vi "HRM-AQN-simulated_read.vi"(8 "error in (no error)":errorcluster, 11 "AQN cluster in":T1) -> (0 "error out":errorcluster, 2 "data":waveform(dbl), 3 "AQN cluster out":T1)   [LabVIEW 2020]
uses:
  HRM-AQN-input_clust.ctl
  <vilib>/measure/NI_MABase.lvlib
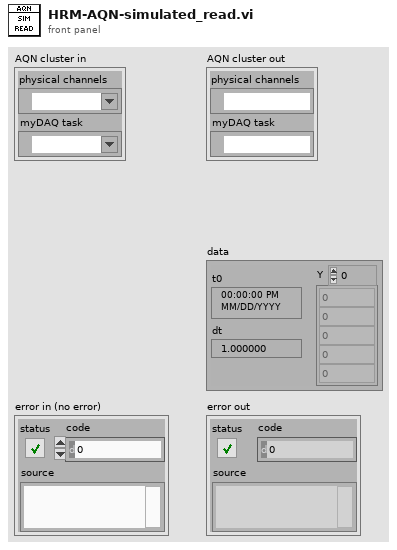
[diagram p1: front panel]
types:
  T1 = typedef "HRM-AQN-input_clust.ctl" = cluster{"physical channels":tag, "myDAQ task":refnum<k21>}
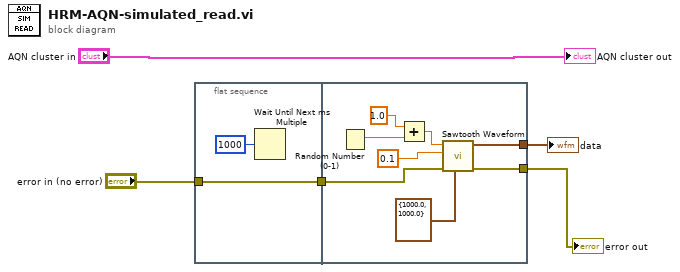
[diagram p0: block diagram]
diagram:
  n1 = flat-sequence {
    tunnel: [w6] -> w2
    tunnel: "error in (no error)" -> [w6]
    tunnel: [w10] -> w4
    tunnel: [w9] -> w3
    tunnel: w2 -> [w8]
    frame #0 {
      n2 = Wait Until Next ms Multiple(millisecond multiple=u32 1000) -> ()  [unwired: 1 out]
    }
    frame #1 {
      n3 = Random Number (0-1)() -> (number: 0 to 1=w13:dbl)
      n4 = Add(x=1.0, y=w13) -> (x+y=w11:dbl)
      n5 = call <vilib>:"Sawtooth Waveform.vi"("sampling info"=cluster{"Fs":dbl, "#s":dbl} {"Fs"=1000.0, "#s"=1000.0}, "error in (no error)"=w8, "amplitude"=0.1, "frequency"=w11) -> ("error out"=w9:errorcluster, "signal out"=w10:waveform(dbl))  [unwired: 6 in]
    }
  }
  "data" <- w4
  "AQN cluster out" <- "AQN cluster in"
  "error out" <- w3
